vi "CPP-GRCclient.vi"(4 "minFlowrate (l/min)":dbl min=0.0 max=360.0 step=1.0 format="%.2f", 5 "Pressure channel":string, 6 "maxFlowrate (l/min)":dbl min=0.0 max=360.0 step=1.0 format="%.2f", 7 "Temperature channel":string, 8 "C_dem:(%)":dbl min=0.0 max=100.0 step=1.0 format="%.2f", 9 "Gas Release System":string, 10 "Q_dem[Total]:(l/min)":dbl min=0.0 step=1.0 format="%.2f", 11 "Mode":T1) -> (0 "errorString":string, 1 "infoString":string, 3 "watchChannels":string[](array[string]))   [LabVIEW 2022 SP3]
uses:
  ADAM Server/Sub VI's/Gas management/CPP/AalborgServerModes.ctl
  Anemometry/Anemometry Sub Vis/Globals/Preference_global.vi
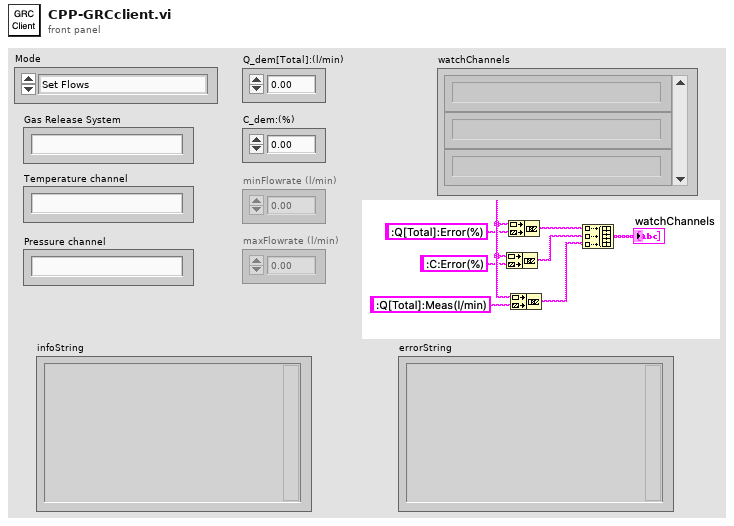
[diagram p1: front panel]
types:
  T1 = typedef "AalborgServerModes.ctl" = enum16{"Set Flows", "Check Flows Are Achievable", "Close All MFCs"}
  T2 = typedef "Server_Comms.ctl" = enum16{"Do Not Link To Server", "Server Link Healthy"}
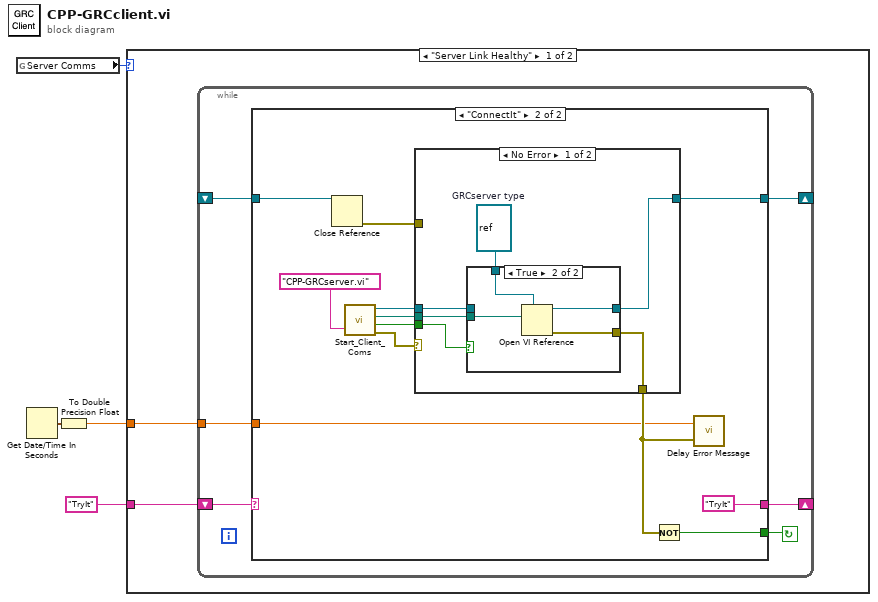
[diagram p0: block diagram]
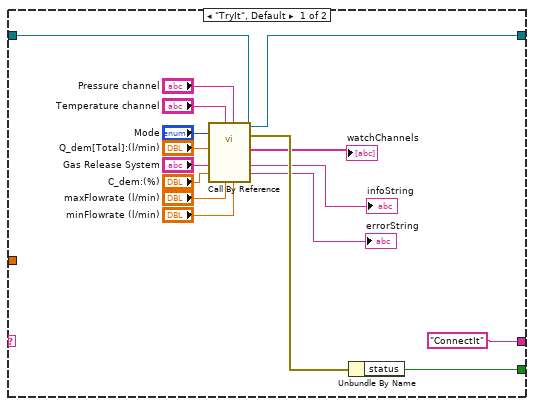
[diagram p2: hidden frame]
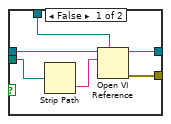
[diagram p3: hidden frame]
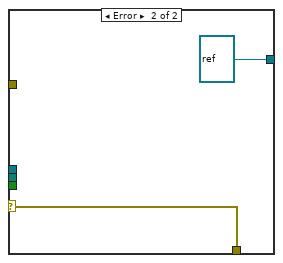
[diagram p4: hidden frame]
diagram:
  n1 = global read "Preference_global.vi" "Server Comms"() -> (w4:T2)
  n2 = Get Date/Time In Seconds() -> (seconds since 1Jan1904=w2:timestamp)
  n3 = To Double Precision Float(number=w2) -> (double precision float=w1:dbl)
  n4 = case shown="\"Server Link Healthy\"" w4 {
    tunnel: "TryIt" -> [w6 _]
    tunnel: w1 -> [w5 _]
    frame "Server Link Healthy" {
      n5 = while {
        shift-left: _ -> [w12]
        shift-right: [w11] -> _
        shift-right: [w9] -> _
        shift-left: w6 -> [w10]
        tunnel: w5 -> [w7]
        stop <- w8 continue-if-true
        n6 = case shown="\"ConnectIt\"" w10 {
          tunnel: w12 -> [w28 w30]
          tunnel: [w27 w36] -> w11
          tunnel: ["ConnectIt" "TryIt"] -> w9
          tunnel: [w16 w34] -> w8
          tunnel: w7 -> [_ w32]
          frame "TryIt", Default {
            n7 = call-by-ref "?"(reference=w28, "minFlowrate (l/min)"="minFlowrate (l/min)", "Pressure channel"="Pressure channel", "maxFlowrate (l/min)"="maxFlowrate (l/min)", "Temperature channel"="Temperature channel", "C:Dem(%)"="C_dem:(%)", "Gas Release System"="Gas Release System", "Q[Total]:Dem(l/min)"="Q_dem[Total]:(l/min)", "Mode"="Mode") -> (reference out=w27:refnum<vi>, error out=w17:errorcluster, "errorString"=→"errorString":string, "infoString"=→"infoString":string, "watchChannels"=→"watchChannels":string[])  [unwired: 2 in]
            n8 = Unbundle By Name(w17) -> ("status"=w16:bool)
          }
          frame "ConnectIt" {
            n9 = Close Reference(reference=w30) -> (error out=w29:errorcluster)  [unwired: 1 in]
            n10 = call "Start_Client_Coms.vi"("VI name to run on server"="CPP-GRCserver.vi") -> ("LabVIEW application reference"=w38:refnum<vi>, "Checked VI name"=w40:path, "Local Call"=w39:bool, "Error cluster"=w31:errorcluster)  [unwired: 1 in]
            n11 = case shown="No Error" w31 {
              selector: w31 -> [_ w58]
              tunnel: w40 -> [w46 _]
              tunnel: w39 -> [w45 _]
              tunnel: w38 -> [w44 _]
              tunnel: [w42 refnum<vi> refnum ("GRCserver type")] -> w36
              tunnel: [w41 w58] -> w33
              tunnel: w29 -> [_ _]
              frame No Error {
                w43 = refnum<vi> refnum  # GRCserver type
                n12 = case shown="True" w45 {
                  tunnel: [w49 w56] -> w42
                  tunnel: w43 -> [w48 w55]
                  tunnel: w46 -> [w50 w54]
                  tunnel: w44 -> [w47 _]
                  tunnel: [w51 w53] -> w41
                  frame False {
                    n13 = Strip Path(path=w50) -> (name=w52:string)  [unwired: 1 out]
                    n14 = Open VI Reference(type specifier VI Refnum (for type only)=w48, application reference (local)=w47, vi path=w52) -> (vi reference=w49:refnum<vi>, error out=w51:errorcluster)  [unwired: 1 in, 2 out]
                  }
                  frame True {
                    n15 = Open VI Reference(type specifier VI Refnum (for type only)=w55, vi path=w54) -> (vi reference=w56:refnum<vi>, error out=w53:errorcluster)  [unwired: 1 in, 3 out]
                  }
                }
              }
              frame Error {
              }
            }
            n16 = Not(x=w33) -> (.not. x?=w34:bool)
            n17 = call "Delay Error Message.vi"("error in (no error)"=w33, "Seconds since 1904"=w32) -> ()  [unwired: 2 in]
          }
        }
      }
    }
    frame "Do Not Link To Server" {
    }
  }
